vi "TEST1.vi"(9 "argv":string[](array[string]), 10 "args":u8) -> ()   [LabVIEW 2011]
panel:
  out "Test output":T1
  out "Status":bool
  out "Input value 2":dbl
  out "Input value 1":dbl
  out "7":bool
  out "6":bool
  out "5":bool
  out "4":bool
  out "3":bool
  out "2":bool
  out "1":bool
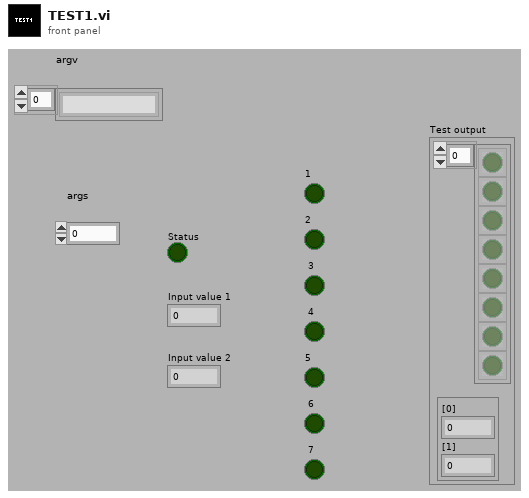
[diagram p1: front panel]
types:
  T1 = cluster{cluster{bool}[], cluster{"[0]":dbl, "[1]":dbl}}
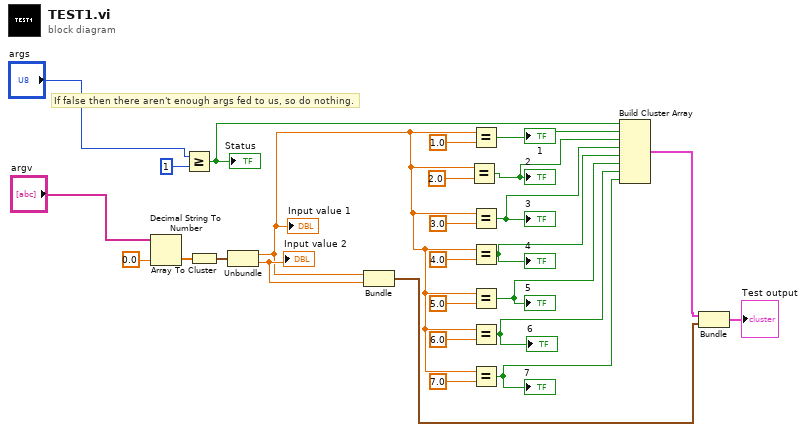
[diagram p0: block diagram]
diagram:
  # "If false then there aren't enough args fed to us, so do nothing."
  n1 = Decimal String To Number(string="argv", default (0L)=0.0 ("default (0 I32)")) -> (number=w24:dbl[])  [unwired: 2 out]
  n2 = Greater Or Equal?(x="args", y=u8 1) -> (x >= y?=w22:bool)
  "Status" <- w22
  n3 = Array To Cluster(array=w24) -> (cluster=w26:cluster{"[0]":dbl, "[1]":dbl})
  n4 = Unbundle(w26) -> ("[0]"=w5:dbl, "[1]"=w21:dbl)
  "Input value 1" <- w5
  "Input value 2" <- w21
  n5 = Bundle("[0]"=w5, "[1]"=w21) -> (w20:cluster{"[0]":dbl, "[1]":dbl})  [unwired: 1 in]
  n6 = Equal?(x=w5, y=2.0) -> (x = y?=w15:bool)
  "2" <- w15
  n7 = Equal?(x=w5, y=1.0) -> (x = y?=w17:bool)
  "1" <- w17
  n8 = Equal?(x=w5, y=3.0) -> (x = y?=w12:bool)
  "3" <- w12
  n9 = Equal?(x=w5, y=4.0) -> (x = y?=w11:bool)
  "4" <- w11
  n10 = Equal?(x=w5, y=5.0) -> (x = y?=w7:bool)
  "5" <- w7
  n11 = Equal?(x=w5, y=6.0) -> (x = y?=w8:bool)
  "6" <- w8
  n12 = Equal?(x=w5, y=7.0) -> (x = y?=w4:bool)
  "7" <- w4
  n13 = Build Cluster Array(w22, w17, w15, w12, w11, w7, w8, w4) -> (w19:cluster{bool}[])
  n14 = Bundle(w19, w20) -> (→"Test output":T1)  [unwired: 1 in]
